vi "test-DC-Motor-Sim-Test2.vi"() -> (3 "All Passed":bool)   [LabVIEW 2019]
uses:
  <vilib>/Rock Robotics/WPI/ThirdParty/JAS_Junk/TrajLib/Trajectory_Library.lvlib
  <vilib>/Analysis/Matrix/Datatypes/RealMatrix.ctl
  <vilib>/Analysis/Matrix/NI_Matrix.lvlib
  <vilib>/Rock Robotics/WPI/ThirdParty/JAS_Junk/TrajLib/DCMotor_GetNEO.vi
panel:
  out "Pos Control Passed":bool
  out "Pos Ctrl":T1(graph)
  out "Error":bool
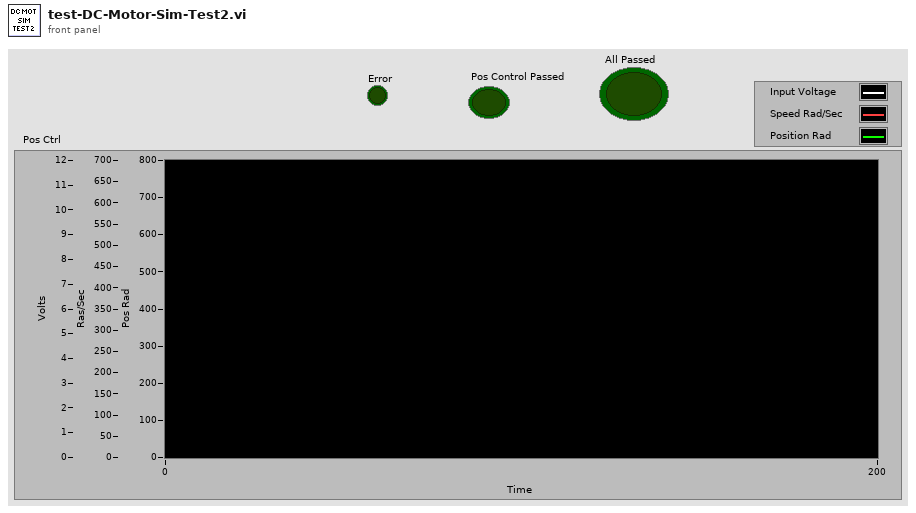
[diagram p1: front panel]
types:
  T1 = cluster{dbl, "Velocity_RadPerSec":dbl, "Position_Rad":dbl}
  T2 = typedef "NI_Matrix.lvlib/RealMatrix.ctl" = dbl[][]
  T3 = typedef "Trajectory_Library.lvlib/DCMOTOR.CTL" = cluster{"nominalVoltage_Volts":dbl, "StallTorque_NM":dbl, "StallCurrent_Amps":dbl, "FreeCurrent_Amps":dbl, "FreeSpeed_RadPerSec":dbl, "R_Ohms":dbl, "KvINV_RadPerSecPerVolt":dbl, "Kt_NMPerAmp":dbl, "L_H":dbl, "Jr_KgM2":dbl}
  T4 = typedef "Trajectory_Library.lvlib/DCMOTOR_SIM.ctl" = cluster{"LinearSystemSim":T5, "GearBox":T3, "Gearing":dbl}
  T5 = typedef "Trajectory_Library.lvlib/LINEAR_SYSTEM_SIM.ctl" = cluster{"m_Plant":T6, "m_X":T2, "m_Y":T2, "m_U":T2, "MeasureStdDev":T2}
  T6 = typedef "Trajectory_Library.lvlib/LINEAR_SYSTEM.ctl" = cluster{"m_A":T2, "m_B":T2, "m_C":T2, "m_D":T2, "States":i32, "Inputs":i32, "Outputs":i32}
  T7 = typedef "Trajectory_Library.lvlib/PID_TUNING.ctl" = cluster{"Kp":dbl, "Ki":dbl, "Kd":dbl, "MaximumIntegral":dbl, "MinimumIntegral":dbl, "IntegralZone":dbl}
  T8 = typedef "Trajectory_Library.lvlib/PID_INPUT_LIMITS.ctl" = cluster{"MaxInput":dbl, "MinInput":dbl, "Continuous":bool}
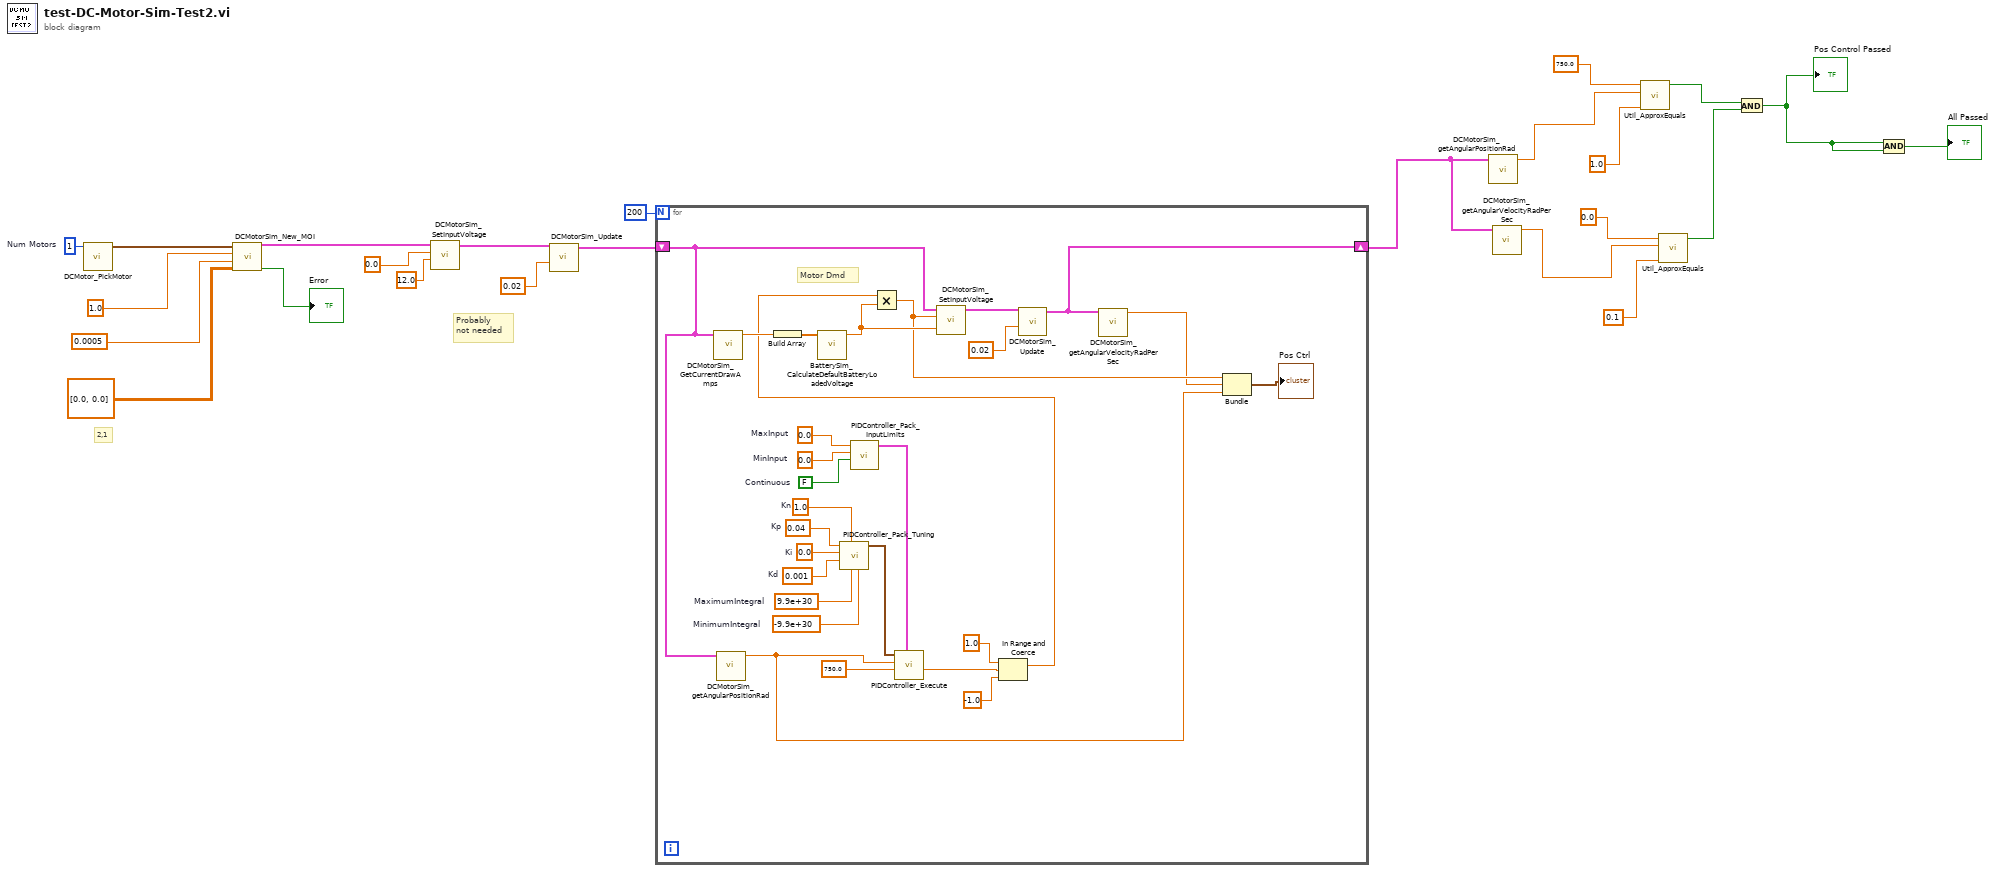
[diagram p0: block diagram]
diagram:
  w24 = 1  # Num Motors
  # "Probably \nnot needed"
  # "2,1"
  n1 = call-poly <vilib>:"DCMotor_PickMotor.vi"("Num Motors"=w24) -> ("DCMOTOR"=w12:T3)  [unwired: 10 in]
  n2 = call <vilib>:"DCMotorSim_New_MOI.vi"("MeasurementStdDev"=T2 [[0.0], [0.0]], "jKgMetersSquared"=0.0005, "Gearing"=1.0, "GearBox"=w12) -> ("Error"=→"Error":bool, "DCMotorSim"=w18:T4)  [unwired: 6 in]
  n3 = call <vilib>:"DCMotorSim_SetInputVoltage.vi"("Battery_Volts"=12.0, "Volts"=0.0, "DCMotorSim"=w18) -> ("out DCMotorSim"=w14:T4)  [unwired: 8 in]
  n4 = call <vilib>:"DCMotorSim_Update.vi"("dT_Seconds"=0.02, "DCMotorSim"=w14) -> ("out DCMotorSim"=w13:T4)  [unwired: 8 in, 1 out]
  n5 = for {
    N: 200 -> [_]
    shift-right: [w43] -> w7
    shift-left: w13 -> [w30]
    w42 = 1.0  # Kn
    w41 = 0.0  # MaxInput
    w40 = 0.0  # MinInput
    w39 = FALSE  # Continuous
    w38 = 0.04  # Kp
    w37 = 0.0  # Ki
    w36 = 0.001  # Kd
    w35 = 9.9e+30  # MaximumIntegral
    w34 = -9.9e+30  # MinimumIntegral
    # "Motor Dmd"
    n6 = call <vilib>:"DCMotorSim_GetCurrentDrawAmps.vi"("DCMotorSim"=w30) -> ("Current_Amps"=w50:dbl)  [unwired: 10 in]
    n7 = call <vilib>:"DCMotorSim_getAngularPositionRad.vi"("DCMotorSim"=w30) -> ("Position_Rad"=w25:dbl)  [unwired: 10 in]
    n8 = Build Array(w50) -> (w51:dbl[])
    n9 = call <vilib>:"BatterySim_CalculateDefaultBatteryLoadedVoltage.vi"("Currents"=w51) -> ("Voltage"=w49:dbl)  [unwired: 10 in]
    n10 = call <vilib>:"PIDController_Pack_Tuning.vi"("MinimumIntegral"=w34, "MaximumIntegral"=w35, "Kn"=w42, "Kd"=w36, "Ki"=w37, "Kp"=w38) -> ("PID Tuning"=w33:T7)  [unwired: 5 in]
    n11 = call <vilib>:"PIDController_Pack_InputLimits.vi"("Continuous"=w39, "MinInput"=w40, "MaxInput"=w41) -> ("PID Input Limits"=w32:T8)  [unwired: 8 in]
    n12 = call <vilib>:"PIDController_Execute.vi"("PID Input Limits"=w32, "SP-SetPoint"=750.0, "PV-Measurement"=w25, "PID Tuning"=w33) -> ("CO-ControlOutput"=w27:dbl)  [unwired: 5 in, 2 out]
    n13 = In Range and Coerce(upper limit=1.0, x=w27, lower limit=-1.0) -> (coerced(x)=w26:dbl)  [unwired: 1 out]
    n14 = Multiply(x=w26, y=w49) -> (x*y=w45:dbl)
    n15 = call <vilib>:"DCMotorSim_SetInputVoltage.vi"("Battery_Volts"=w49, "Volts"=w45, "DCMotorSim"=w30) -> ("out DCMotorSim"=w48:T4)  [unwired: 8 in]
    n16 = call <vilib>:"DCMotorSim_Update.vi"("dT_Seconds"=0.02, "DCMotorSim"=w48) -> ("out DCMotorSim"=w43:T4)  [unwired: 8 in, 1 out]
    n17 = call <vilib>:"DCMotorSim_getAngularVelocityRadPerSec.vi"("DCMotorSim"=w43) -> ("Velocity_RadPerSec"=w44:dbl)  [unwired: 10 in]
    n18 = Bundle(w45, "Velocity_RadPerSec"=w44, "Position_Rad"=w25) -> (→"Pos Ctrl":T1)  [unwired: 1 in]
  }
  n19 = call <vilib>:"DCMotorSim_getAngularPositionRad.vi"("DCMotorSim"=w7) -> ("Position_Rad"=w8:dbl)  [unwired: 10 in]
  n20 = call <vilib>:"DCMotorSim_getAngularVelocityRadPerSec.vi"("DCMotorSim"=w7) -> ("Velocity_RadPerSec"=w4:dbl)  [unwired: 10 in]
  n21 = call <vilib>:"Util_ApproxEquals.vi"("Tolerance"=1.0, "Value 2"=w8, "Value 1"=750.0 ("y")) -> ("ApproxEquals"=w3:bool)  [unwired: 8 in]
  n22 = call <vilib>:"Util_ApproxEquals.vi"("Tolerance"=0.1, "Value 2"=w4, "Value 1"=0.0 ("y")) -> ("ApproxEquals"=w2:bool)  [unwired: 8 in]
  n23 = And(x=w3, y=w2) -> (x .and. y?=w1:bool)
  "Pos Control Passed" <- w1
  n24 = And(x=w1, y=w1) -> (x .and. y?=→"All Passed":bool)
